vi "Contains Key.vi"(8 "error in":errorcluster, 10 "Key":string, 11 "Section in":refnum<class "Section.lvclass">) -> (0 "error out":errorcluster, 1 "Index":i32, 2 "Contains Key?":bool, 3 "Section out":refnum<class "Section.lvclass">)   [LabVIEW 2019, in "Electronic Datasheet.lvlib" / "Section.lvclass"]
uses:
  Section.lvclass
  Section.lvclass/Section.ctl
  Keyname/Key Name.lvclass
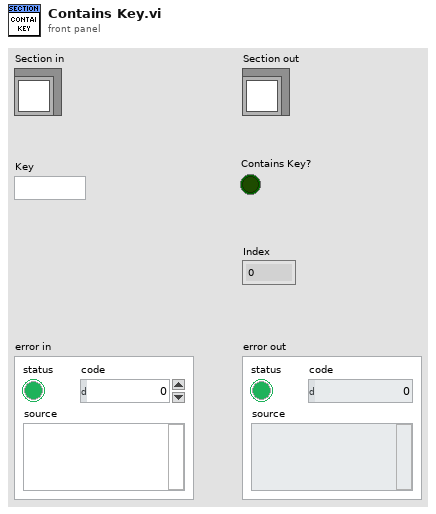
[diagram p1: front panel]
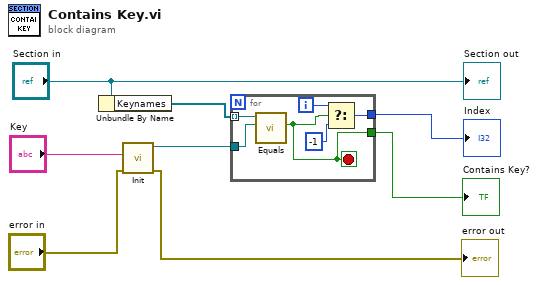
[diagram p0: block diagram]
diagram:
  n1 = Unbundle By Name("Section in") -> ("Keynames"=w7:refnum<class "Key Name.lvclass">[])
  n2 = call "Init.vi"("error in"="error in", "Key Name"="Key") -> ("error out"=→"error out":errorcluster, "Key Name out"=w5:refnum<class "Key Name.lvclass">)  [unwired: 8 in]
  n3 = for {
    tunnel: w7 -> [w14] mode=indexing
    tunnel: [w11] -> w3
    tunnel: w5 -> [w13]
    tunnel: [w9] -> w4
    i -> [w12]
    stop <- w9 stop-if-true
    n4 = call "Equals.vi"("Keyname"=w13, "Keyname in"=w14) -> ("Equal?"=w9:bool)  [unwired: 8 in, 1 out]
    n5 = Select(t=w12, s=w9, f=-1) -> (s? t:f=w11:i32)
  }
  "Contains Key?" <- w4
  "Index" <- w3
  "Section out" <- "Section in"
